vi "find_StdObject_by_Name.vi"(10 "std_name":string, 11 "StdObj Array in":refnum<class "Standard.lvclass">[](array[class])) -> (0 "index of Object in Array":i32, 1 "found?":bool, 2 "found StdObj out":refnum<class "Standard.lvclass">, 3 "StdObj Array out":refnum<class "Standard.lvclass">[](array[class]))   [LabVIEW 2018]
doc: "Find the correct StdObject by the Name of the Standard"
uses:
  Classes/Standard/Standard.lvclass
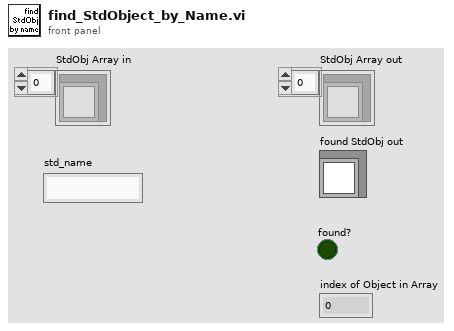
[diagram p1: front panel]
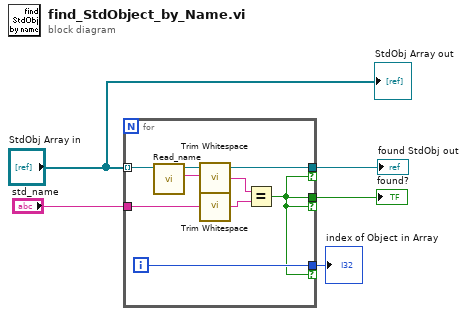
[diagram p0: block diagram]
diagram:
  n1 = for {
    tunnel: "std_name" -> [w13]
    tunnel: [w10] -> w4 if=w6
    tunnel: "StdObj Array in" -> [w8] mode=indexing
    tunnel: [w6] -> w3 if=w6
    tunnel: [w7] -> w1 if=w6
    i -> [w7]
    n2 = call-dynamic "Read_name.vi"("Standard in"=w8) -> ("standard name"=w9:string, "Standard out"=w10:refnum<class "Standard.lvclass">)  [unwired: 8 in, 1 out]
    n3 = call <vilib>:"Trim Whitespace.vi"("string"=w9) -> ("trimmed string"=w12:string)  [unwired: 1 in]
    n4 = call <vilib>:"Trim Whitespace.vi"("string"=w13) -> ("trimmed string"=w11:string)  [unwired: 1 in]
    n5 = Equal?(x=w12, y=w11) -> (x = y?=w6:bool)
  }
  "found StdObj out" <- w4
  "found?" <- w3
  "index of Object in Array" <- w1
  "StdObj Array out" <- "StdObj Array in"
